vi "Close Sysdef Refs for IP Set.vi"(8 "error in (no error)":errorcluster, 10 "Sysdef":refnum<k24>, 11 "Targets":refnum<k24>[](array[refnum])) -> (0 "error out":errorcluster)   [LabVIEW 2011]
uses:
  NationalInstruments.VeriStand.SystemDefinitionAPI
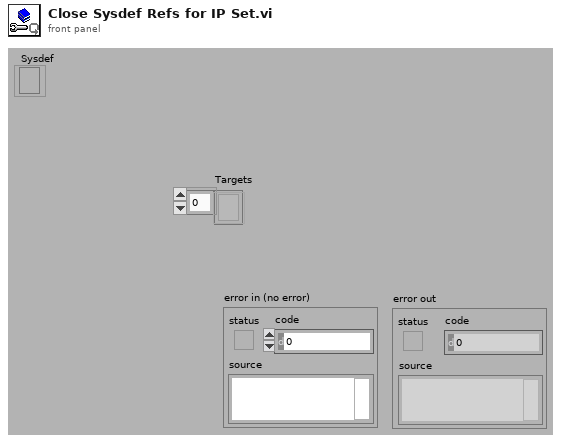
[diagram p1: front panel]
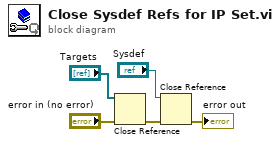
[diagram p0: block diagram]
diagram:
  n1 = Close Reference(reference="Targets", error in (no error)="error in (no error)") -> (error out=w5:errorcluster)
  n2 = Close Reference(reference="Sysdef", error in (no error)=w5) -> (error out=→"error out":errorcluster)
